vi "16_Bit_to_Byte_String.vi"(2 "Radix Format":enum32{"include 0x Radix", "No Radix"}(radio), 3 "16 bit in":u16 format="%x") -> (0 "LSB OUT":string, 1 "MSB OUT":string)   [LabVIEW 2011]
doc: "This VI converts a 16 bit integer to two 8 bit hex strings. The USB-DAQ Mnemonic commands use hexadecimal strings including the radix (e.g. \"0xAF\"). This VI will make format the two 8 bit strings as required by \"Run_Mnemonic_Command.vi\"."
panel:
  in  "Vexc Input":dbl min=0.0 max=5.5
  # "Input"
  # "Output"
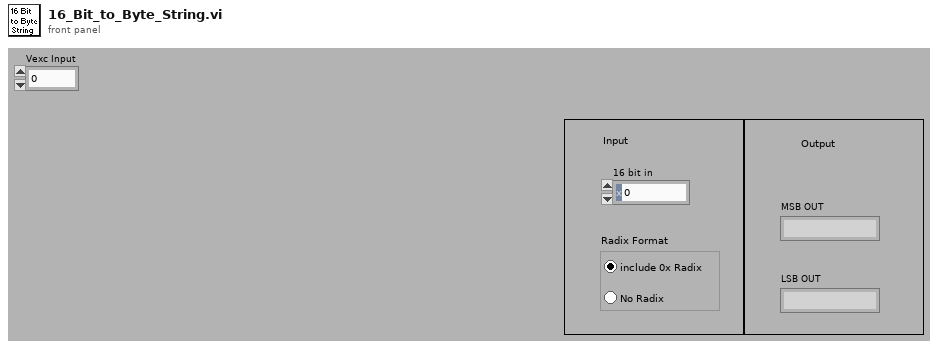
[diagram p1: front panel]
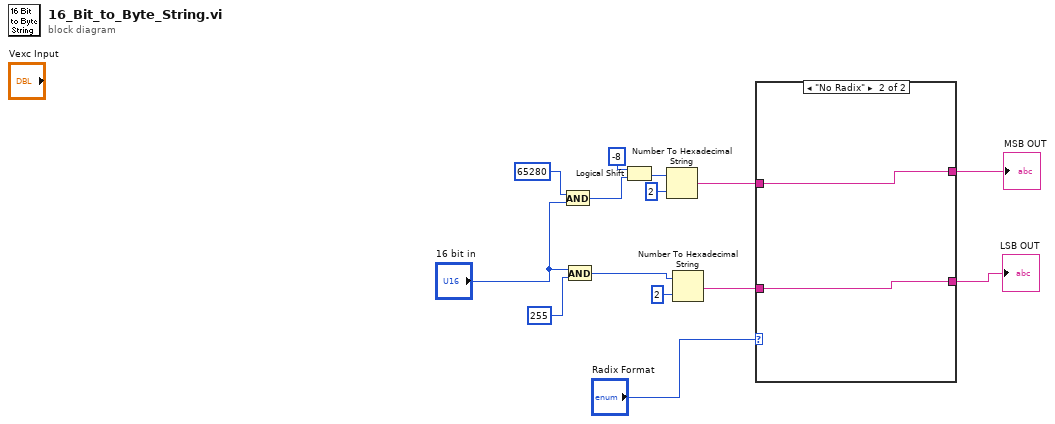
[diagram p0: block diagram]
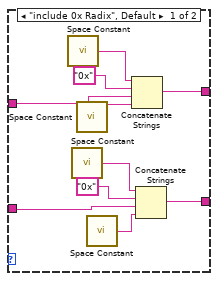
[diagram p2: hidden frame]
diagram:
  n1 = And(x=u16 65280, y="16 bit in") -> (x .and. y?=w11:u16)
  n2 = And(x="16 bit in", y=u16 255 ("x")) -> (x .and. y?=w12:u16)
  n3 = Logical Shift(y=i16 -8 ("x"), x=w11) -> (x << y=w10:u16)
  n4 = Number To Hexadecimal String(1:i16 2 ("width (-)"), 2:w10) -> (0:w9:string)
  n5 = Number To Hexadecimal String(1:i16 2 ("width (-)"), 2:w12) -> (0:w6:string)
  n6 = case shown="\"No Radix\"" "Radix Format" {
    tunnel: w9 -> [w15 w26]
    tunnel: [w17 w25] -> w8
    tunnel: [w16 w26] -> w7
    tunnel: w6 -> [w18 w25]
    frame "include 0x Radix", Default {
      n7 = call <vilib>:"Space Constant.vi"() -> ("String"=w20:string)
      n8 = call <vilib>:"Space Constant.vi"() -> ("String"=w19:string)
      n9 = call <vilib>:"Space Constant.vi"() -> ("String"=w22:string)
      n10 = call <vilib>:"Space Constant.vi"() -> ("String"=w21:string)
      n11 = Concatenate Strings(w20, "0x" ("string"), w15, w22) -> (w16:string)
      n12 = Concatenate Strings(w19, "0x" ("string"), w18, w21) -> (w17:string)
    }
    frame "No Radix" {
    }
  }
  "MSB OUT" <- w7
  "LSB OUT" <- w8
